vi "W_Open_result_file_plotter.vi"   [LabVIEW 2010]
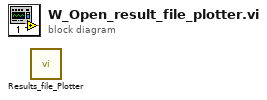
[diagram p0: block diagram]
diagram:
  n1 = call "Results_file_Plotter.vi"() -> ()  [unwired: 20 in]
